vi "Line Detector Initial Guess from Peak Findervi.vi"(6 "Peak finder guess":dbl[](array[numeric]), 10 "Signal":cdb[](array[numeric])) -> (3 "Initial guess":dbl[](array[numeric]))   [LabVIEW 2016]
panel:
  # "F0\n\nAmpl\n\nWidth"
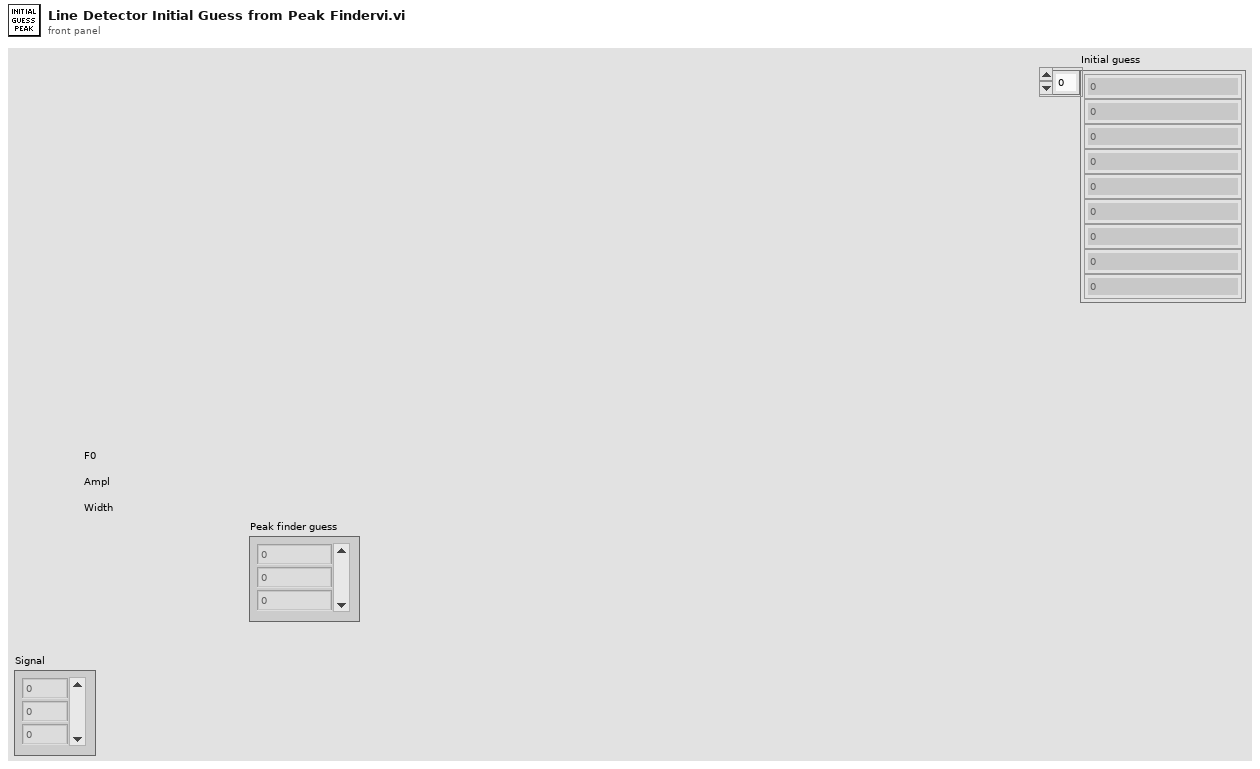
[diagram p1: front panel]
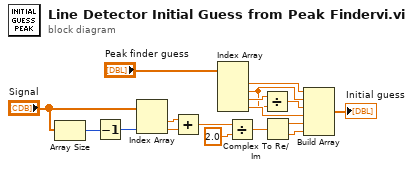
[diagram p0: block diagram]
diagram:
  n1 = Array Size(array="Signal") -> (size(s)=w16:i32)
  n2 = Decrement(x=w16) -> (x-1=w15:i32)
  n3 = Index Array(array="Signal", index #2=w15) -> (element #1=w14:cdb, element #2=w13:cdb)  [unwired: 1 in]
  n4 = Add(x=w14, y=w13) -> (x+y=w12:cdb)
  n5 = Index Array(array="Peak finder guess") -> (element #1=w9:dbl, element #2=w2:dbl, element #3=w3:dbl, element #4=w5:dbl)  [unwired: 4 in]
  n6 = Divide(x=w12, y=2.0) -> (x/y=w8:cdb)
  n7 = Divide(x=w3, y=w2) -> (x/y=w1:dbl)
  n8 = Complex To Re/Im(x + iy=w8) -> (x=w11:dbl, y=w10:dbl)
  n9 = Build Array(w9, w2, w1, w5, w11, w10) -> (→"Initial guess":dbl[])
